vi "ReaderDaemon.vi"(8 "error in (no error)":errorcluster, 9 "Stop command reference":refnum<data-value>, 10 "Variant Queue":T1, 11 "Reader Endpoint":refnum<k21>) -> ()   [LabVIEW 2011, in "NetworkStreamReader.lvclass"]
doc: "Daemon (running in the background) which consistently checks the reader endpoint to see if a new value is available, and then passes it into the internal queue of the NetworkStreamReader if data is available."
uses:
  NetworkStreamReader.lvclass
  Shared/messageQueue.ctl
  Shared/message.ctl
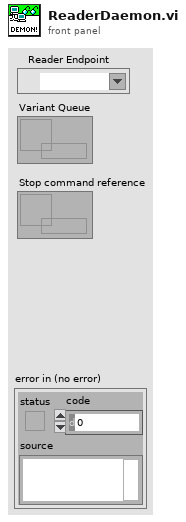
[diagram p1: front panel]
types:
  T1 = typedef "messageQueue.ctl" = refnum<queue>
  T2 = typedef "message.ctl" = cluster{"Data":variant, "Time since start (s)":dbl}
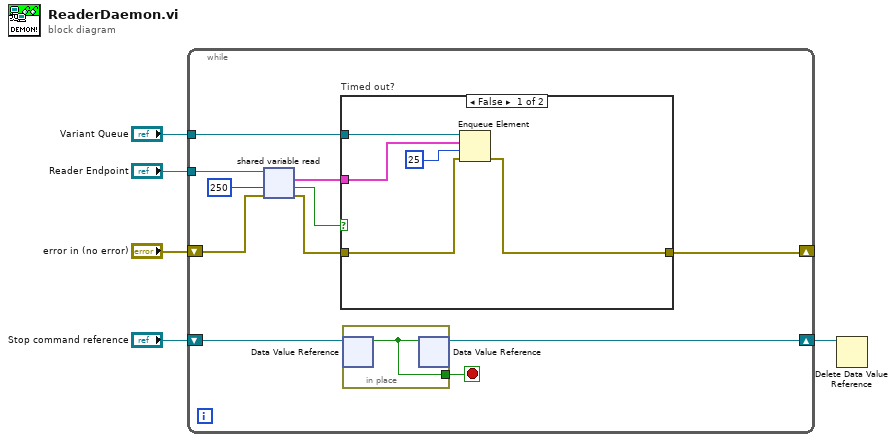
[diagram p0: block diagram]
diagram:
  n1 = while {
    tunnel: "Reader Endpoint" -> [w16]
    tunnel: "Variant Queue" -> [w11]
    shift-right: [w10] -> _
    shift-left: "error in (no error)" -> [w15]
    shift-right: [w7] -> w3
    shift-left: "Stop command reference" -> [w9]
    stop <- w8 stop-if-true
    n2 = shared-variable-read(w16, w15, 250 ("timeout in ms (-1)")) -> (w13:errorcluster, w12:bool, w6:T2)  [unwired: 1 out]
    n3 = case "Timed out?" shown="False" w12 {
      tunnel: w13 -> [w20 w23]
      tunnel: w11 -> [w22 _]
      tunnel: [w19 w23] -> w10
      tunnel: w6 -> [w18 _]
      frame False {
        n4 = Enqueue Element(queue=w22, element=w18, timeout in ms (-1)=25, error in (no error)=w20) -> (error out=w19:errorcluster)  [unwired: 2 out]
      }
      frame True {
      }
    }
    n5 = in-place {
      in-place-border: [w17] -> w8
      n6 = in-place-dvr #1(w9) -> (w17:bool)  [unwired: 1 out]
      n7 = in-place-dvr #1(w17) -> (w7:refnum<data-value>)  [unwired: 1 out]
    }
  }
  n8 = Delete Data Value Reference(data value reference=w3) -> ()  [unwired: 1 in, 2 out]
